vi "Calculate_x2dot.vi"(6 "a4":dbl, 7 "x1_norm":dbl, 9 "a3":dbl, 10 "a5":dbl, 11 "x2":dbl) -> (3 "x2dot":dbl)   [LabVIEW 2013]
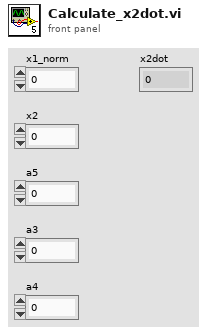
[diagram p1: front panel]
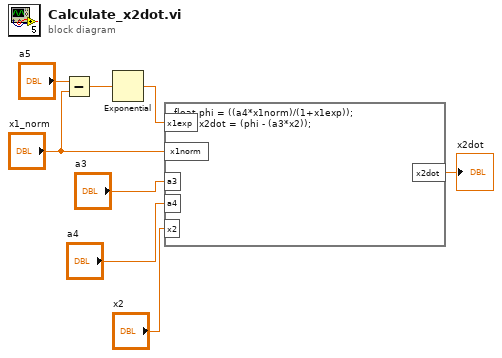
[diagram p0: block diagram]
diagram:
  n1 = Subtract(x="a5", y="x1_norm") -> (x-y=w2:dbl)
  n2 = Exponential(1:w2) -> (0:w3:dbl)
  n3 = formula code="float phi = ((a4*x1norm)/(1+x1exp));\nfloat x2dot = (phi - (a3*x2));"("a3"="a3", "a4"="a4", "x1norm"="x1_norm", "x1exp"=w3, "x2"="x2") -> ("x2dot"=→"x2dot":dbl)
